vi "Fill Out Project VIs .vi"(7 "Project Member Data":string[][](array[string]), 8 "error in (no error)":errorcluster, 11 "NI_report in":refnum<class "NI_report.lvclass">) -> (0 "error out":errorcluster, 3 "NI_report out":refnum<class "NI_report.lvclass">)   [LabVIEW 2014]
uses:
  <vilib>/Utility/NIReport.llb/NI_report.lvclass
  <vilib>/addons/_office/excel.llb/Excel Easy Table (str).vi
  <vilib>/Utility/NIReport.llb/Excel/NI_Excel.lvclass
  <vilib>/addons/_office/NI_ReportGenerationToolkit.lvlib
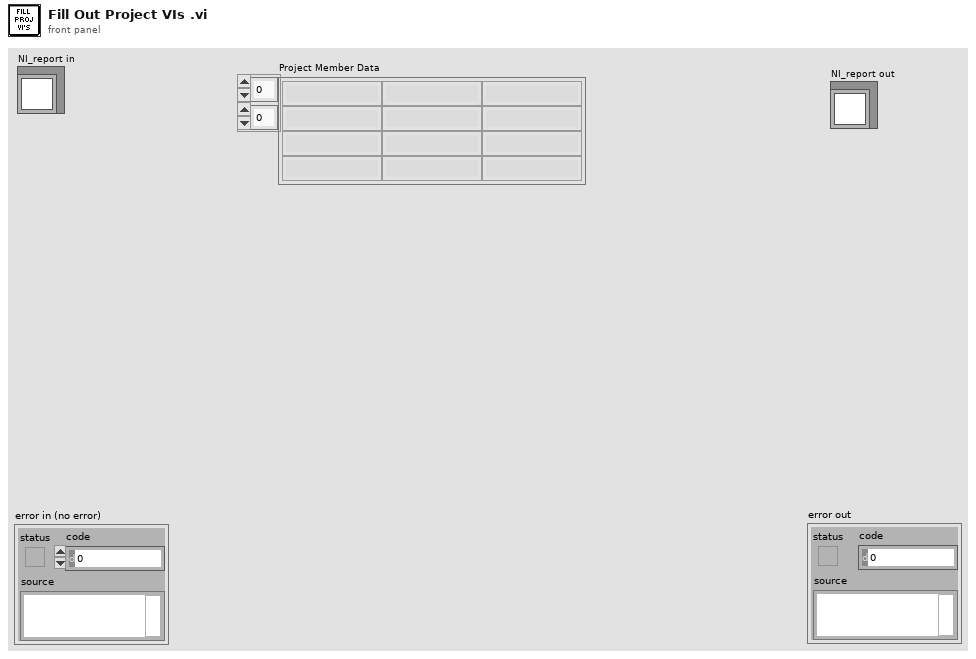
[diagram p1: front panel]
types:
  T1 = cluster{"on/off":bool, "weight":i32, "color":u32}
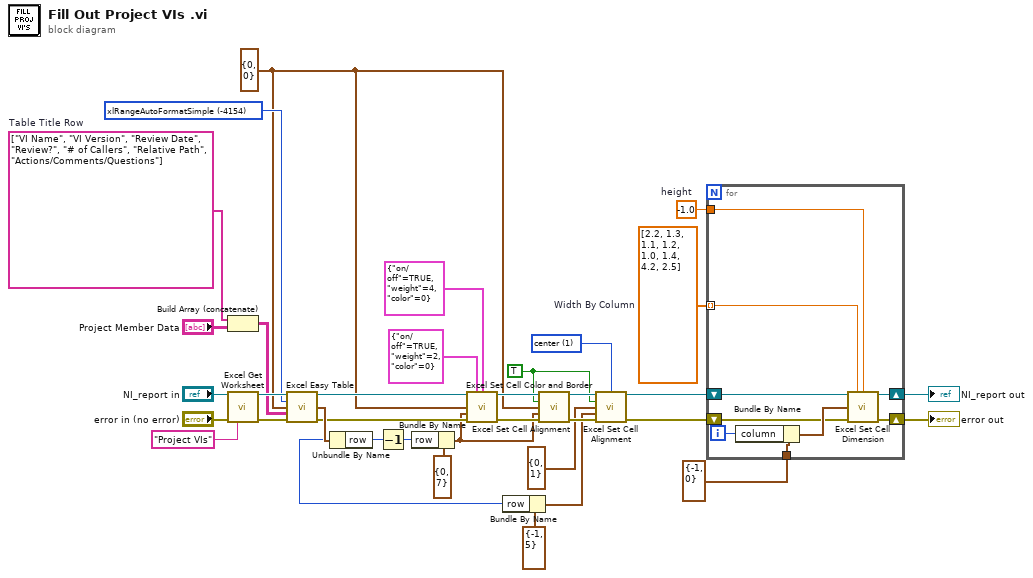
[diagram p0: block diagram]
diagram:
  w7 = 1 items=["left", "center", "right"] ("horizontal alignment (left)")
  w14 = -1.0  # height
  w19 = dbl[] [2.2, 1.3, 1.1, 1.2, 1.0, 1.4, 4.2, 2.5]  # Width By Column
  w8 = TRUE ("wrap text? (F)")
  w26 = string[] ["VI Name", "VI Version", "Review Date", "Review?", "# of Callers", "Relative Path", "Actions/Comments/Questions"]  # Table Title Row
  w27 = -4154 items=["xlRangeAutoFormat3DEffects1"=13, "xlRangeAutoFormat3DEffects2"=14, "xlRangeAutoFormatAccounting1"=4, "xlRangeAutoFormatAccounting2"=5, "xlRangeAutoFormatAccounting3"=6, "xlRangeAutoFormatAccounting4"=17, "xlRangeAutoFormatClassic1"=1, "xlRangeAutoFormatClassic2"=2, "xlRangeAutoFormatClassic3"=3, "xlRangeAutoFormatColor1"=7, "xlRangeAutoFormatColor2"=8, "xlRangeAutoFormatColor3"=9, "xlRangeAutoFormatList1"=10, "xlRangeAutoFormatList2"=11, "xlRangeAutoFormatList3"=12, "xlRangeAutoFormatLocalFormat1"=15, "xlRangeAutoFormatLocalFormat2"=16, "xlRangeAutoFormatLocalFormat3"=19, "xlRangeAutoFormatLocalFormat4"=20, "xlRangeAutoFormatReport1"=21, "xlRangeAutoFormatReport2"=22, "xlRangeAutoFormatReport3"=23, "xlRangeAutoFormatReport4"=24, "xlRangeAutoFormatReport5"=25, "xlRangeAutoFormatReport6"=26, "xlRangeAutoFormatReport7"=27, "xlRangeAutoFormatReport8"=28, "xlRangeAutoFormatReport9"=29, "xlRangeAutoFormatReport10"=30, "xlRangeAutoFormatClassicPivotTable"=31, "xlRangeAutoFormatTable1"=32, "xlRangeAutoFormatTable2"=33, "xlRangeAutoFormatTable3"=34, "xlRangeAutoFormatTable4"=35, "xlRangeAutoFormatTable5"=36, "xlRangeAutoFormatTable6"=37, "xlRangeAutoFormatTable7"=38, "xlRangeAutoFormatTable8"=39, "xlRangeAutoFormatTable9"=40, "xlRangeAutoFormatTable10"=41, "xlRangeAutoFormatPTNone"=42, "xlRangeAutoFormatNone"=-4142, "xlRangeAutoFormatSimple"=-4154] ("auto format (none)")
  w18 = cluster{"row":i32, "column":i32} {"row"=0, "column"=0} ("start (-1, -1)")
  n1 = Build Array (concatenate)(w26, "Project Member Data") -> (w24:string[][])
  n2 = call <vilib>:"Excel Get Worksheet.vi"("report in"="NI_report in", "error in (no error)"="error in (no error)", "name (\"\")"="Project VIs" ("name (\"\")")) -> ("report out"=w32:refnum<class "NI_report.lvclass">, "error out"=w33:errorcluster)  [unwired: 11 in]
  n3 = call-poly <vilib>:"Excel Easy Table.vi"("report in"=w32, "auto format (none)"=w27, "start (0, 0)"=w18, "text data"=w24, "error in (no error)"=w33) -> ("report out"=w30:refnum<class "NI_report.lvclass">, "next cell bottom-left"=w22:cluster{"row":i32, "column":i32}, "error out"=w16:errorcluster)  [unwired: 6 in, 2 out]
  n4 = Unbundle By Name(w22) -> ("row"=w3:i32)
  n5 = Decrement(x=w3) -> (x-1=w21:i32)
  n6 = Bundle By Name(cluster=cluster{"row":i32, "column":i32} {"row"=0, "column"=7} ("start (-1, -1)"), "row"=w21) -> (w9:cluster{"row":i32, "column":i32})
  n7 = call <vilib>:"Excel Set Cell Color and Border.vi"("report in"=w30, "inside border"=T1 {"on/off"=TRUE, "weight"=2, "color"=0}, "outside border"=T1 {"on/off"=TRUE, "weight"=4, "color"=0}, "start (-1, -1)"=w18, "end (-1, -1)"=w9, "error in (no error)"=w16) -> ("report out"=w23:refnum<class "NI_report.lvclass">, "error out"=w15:errorcluster)  [unwired: 8 in]
  n8 = Bundle By Name(cluster=cluster{"row":i32, "column":i32} {"row"=-1, "column"=5} ("start (-1, -1)"), "row"=w3) -> (w4:cluster{"row":i32, "column":i32})
  n9 = call <vilib>:"Excel Set Cell Alignment.vi"("report in"=w23, "wrap text? (F)"=w8, "start (-1, -1)"=w18, "end (-1, -1)"=w9, "error in (no error)"=w15) -> ("report out"=w13:refnum<class "NI_report.lvclass">, "error out"=w11:errorcluster)  [unwired: 9 in]
  n10 = call <vilib>:"Excel Set Cell Alignment.vi"("report in"=w13, "horizontal alignment (left)"=w7, "wrap text? (F)"=w8, "start (-1, -1)"=cluster{"row":i32, "column":i32} {"row"=0, "column"=1}, "end (-1, -1)"=w4, "error in (no error)"=w11) -> ("report out"=w12:refnum<class "NI_report.lvclass">, "error out"=w10:errorcluster)  [unwired: 8 in]
  n11 = for {
    tunnel: w19 -> [w42] mode=indexing
    tunnel: cluster{"row":i32, "column":i32} {"row"=-1, "column"=0} ("start (-1, -1)") -> [w41]
    shift-right: [w43] -> w2
    shift-left: w12 -> [w44]
    shift-right: [w40] -> w1
    shift-left: w10 -> [w37]
    tunnel: w14 -> [w36]
    i -> [w38]
    n12 = Bundle By Name(cluster=w41, "column"=w38) -> (w39:cluster{"row":i32, "column":i32})
    n13 = call <vilib>:"Excel Set Cell Dimension.vi"("report in"=w44, "width (-1)"=w42, "height (-1)"=w36, "start (-1, -1)"=w39, "error in (no error)"=w37) -> ("report out"=w43:refnum<class "NI_report.lvclass">, "error out"=w40:errorcluster)  [unwired: 9 in]
  }
  "error out" <- w1
  "NI_report out" <- w2
